vi "element_editor_hydrolysis_initial.vi"(9 "Env. Dir":refnum<vi>, 10 "Env. Ready?":refnum<vi>, 11 "Break":refnum<vi>) -> ()   [LabVIEW 2019]
uses:
  lib/libSimulationControl/libSimulationControl.lvlib
panel:
  # "*******************************************************************\nBiogas Plant Control\n\nAuthor: Paul Zügel\nGCSC-Frankfurt am Main 2020\n\n*******************************************************************"
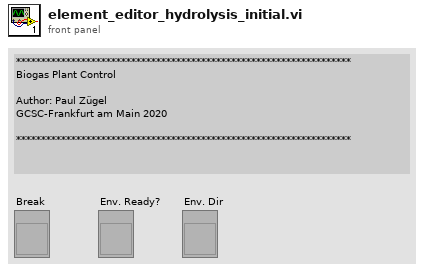
[diagram p1: front panel]
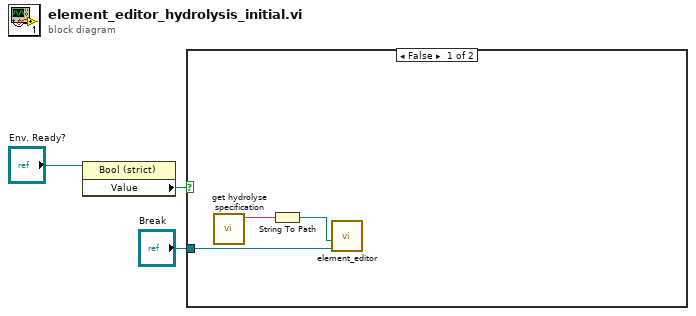
[diagram p0: block diagram]
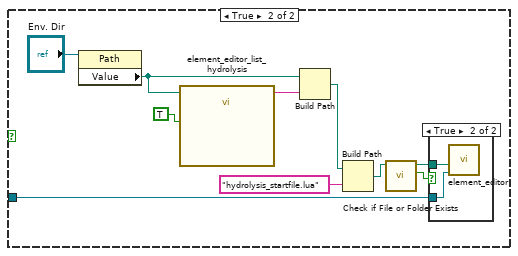
[diagram p2: hidden frame]
diagram:
  n1 = property class="Bool (strict)"(reference="Env. Ready?") -> ("Value"=w2:bool)  [unwired: 1 in, 2 out]
  n2 = case shown="False" w2 {
    tunnel: "Break" -> [w6 w12]
    frame False {
      n3 = call "get hydrolyse specification.vi"() -> ("function return"=w5:string)  [unwired: 10 in, 1 out]
      n4 = String To Path(string=w5) -> (path=w4:path)
      n5 = call "element_editor.vi"("Break"=w6, "LUA Specification File"=w4) -> ()  [unwired: 5 in, 1 out]
    }
    frame True {
      n6 = property on="Property Node" class="Path"(reference="Env. Dir") -> ("Value"=w15:path)  [unwired: 1 in, 2 out]
      n7 = call "element_editor_list_hydrolysis.vi"("Allow all?"=TRUE, "path"=w15) -> ("Value"=w14:string)  [unwired: 6 in, 3 out]
      n8 = Build Path(base path=w15, name or relative path=w14) -> (appended path=w10:path)
      n9 = Build Path(base path=w10, name or relative path="hydrolysis_startfile.lua") -> (appended path=w8:path)
      n10 = call <vilib>:"Check if File or Folder Exists.vi"("path"=w8) -> ("file or folder exists?"=w13:bool, "dup path"=w7:path)  [unwired: 8 in, 1 out]
      n11 = case shown="True" w13 {
        tunnel: w12 -> [_ w18]
        tunnel: w7 -> [_ w17]
        frame False {
        }
        frame True {
          n12 = call "element_editor.vi"("Break"=w18, "LUA Specification File"=w17) -> ()  [unwired: 5 in, 1 out]
        }
      }
    }
  }
